vi "Create Histogram Data.vi"(0 "VISA resource name":refnum<visa-resource-name>, 5 "Number of Item (50)":u32=50, 7 "Width (5)":u32=5, 9 "Array Data":dbl[](array[numeric]) format="%.2f", 11 "error in (no error)":errorcluster) -> (4 "VISA resource name out":refnum<visa-resource-name>, 10 "Histogram Data":dbl[](array[numeric]) format="%.2f", 15 "error out":errorcluster)   [LabVIEW 2013, in "Yokogawa.lvlib" / "Yokogawa PZ4000.lvlib"]
doc: "Create Histogram Data From 1DArray Data"
uses:
  Yokogawa PZ4000.lvlib
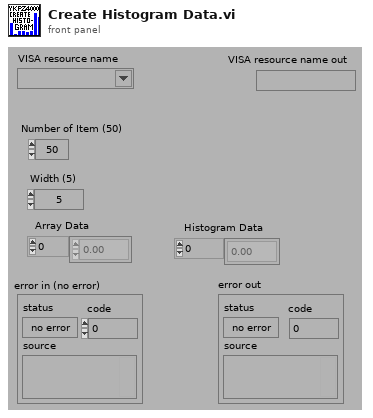
[diagram p1: front panel]
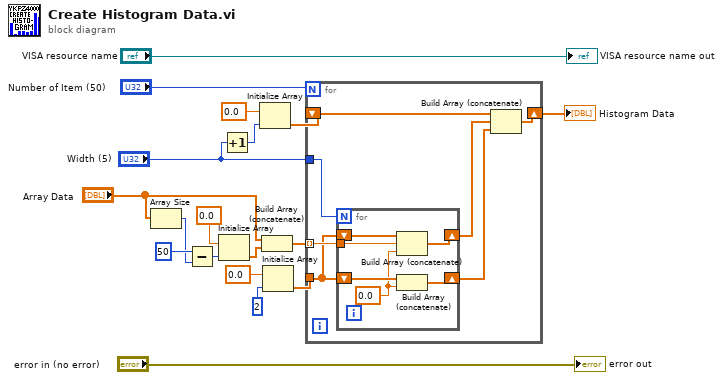
[diagram p0: block diagram]
diagram:
  n1 = Array Size(array="Array Data") -> (size(s)=w4:i32)
  n2 = Subtract(x=50, y=w4) -> (x-y=w9:i32)
  n3 = Initialize Array(0.0, w9) -> (w7:dbl[])
  n4 = Increment(x="Width (5)") -> (x+1=w15:u32)
  n5 = Initialize Array(0.0, w15) -> (w13:dbl[])
  n6 = Build Array (concatenate)("Array Data", w7) -> (w6:dbl[])
  n7 = Initialize Array(0.0, 2) -> (w12:dbl[])
  n8 = for {
    N: "Number of Item (50)" -> [_]
    shift-right: [w24] -> w16
    shift-left: w13 -> [w25]
    tunnel: "Width (5)" -> [w23]
    tunnel: w6 -> [w22] mode=indexing
    tunnel: w12 -> [w19]
    n9 = for {
      N: w23 -> [_]
      shift-right: [w29] -> w21
      shift-left: w19 -> [w30]
      tunnel: w22 -> [w31]
      shift-right: [w27] -> w20
      shift-left: w19 -> [w28]
      w26 = 0.0
      n10 = Build Array (concatenate)(w30, w31, w26) -> (w29:dbl[])
      n11 = Build Array (concatenate)(w28, w26) -> (w27:dbl[])
    }
    n12 = Build Array (concatenate)(w25, w21, w20) -> (w24:dbl[])
  }
  "Histogram Data" <- w16
  "error out" <- "error in (no error)"
  "VISA resource name out" <- "VISA resource name"
